vi "Distance.vi"(8 "error in (no error)":errorcluster, 10 "Galaxy in 2":refnum<class "Galaxy.lvclass">, 11 "Galaxy in":refnum<class "Galaxy.lvclass">) -> (0 "error out":errorcluster, 2 "Numeric":u64)   [LabVIEW 2020, in "Galaxy.lvclass"]
uses:
  Galaxy.lvclass
  Galaxy.lvclass/Galaxy.ctl
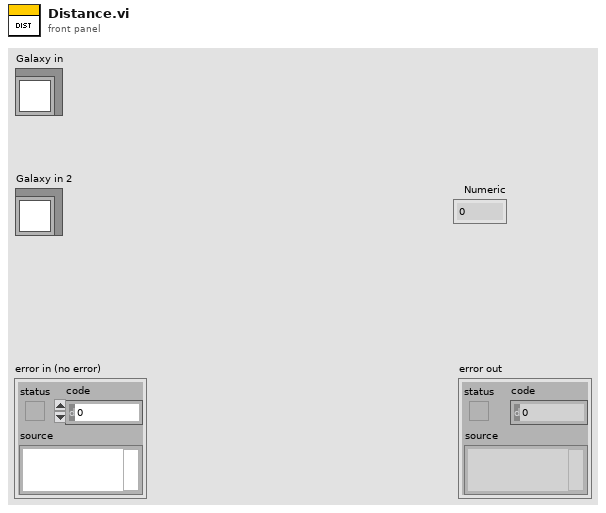
[diagram p1: front panel]
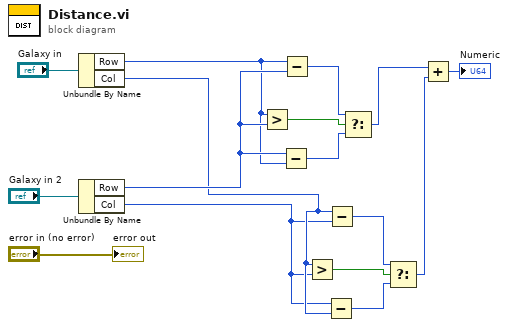
[diagram p0: block diagram]
diagram:
  n1 = Unbundle By Name("Galaxy in") -> ("Row"=w10:u64, "Col"=w3:u64)
  n2 = Unbundle By Name("Galaxy in 2") -> ("Row"=w11:u64, "Col"=w1:u64)
  n3 = Greater?(x=w10, y=w11) -> (0:w12:bool)
  n4 = Subtract(x=w11, y=w10) -> (x-y=w9:u64)
  n5 = Subtract(x=w10, y=w11) -> (x-y=w8:u64)
  n6 = Greater?(x=w3, y=w1) -> (0:w4:bool)
  n7 = Subtract(x=w1, y=w3) -> (x-y=w5:u64)
  n8 = Subtract(x=w3, y=w1) -> (x-y=w6:u64)
  n9 = Select(t=w8, s=w12, f=w9) -> (s? t:f=w7:u64)
  n10 = Select(t=w6, s=w4, f=w5) -> (s? t:f=w2:u64)
  n11 = Add(x=w7, y=w2) -> (x+y=→"Numeric":u64)
  "error out" <- "error in (no error)"
